vi "test Create Number of Tags.vi"(8 "error in (no error)":errorcluster, 11 "TestCase in":refnum<class "TagTests.lvclass">) -> (0 "error out":errorcluster, 3 "TestCase out":refnum<class "TagTests.lvclass">)   [LabVIEW 2014, in "TagTests.lvclass"]
uses:
  TagTests.lvclass
  <vilib>/addons/_JKI Toolkits/VI Tester/TestCase.llb/TestCase.lvclass
  SPLAT/Tag.lvclass
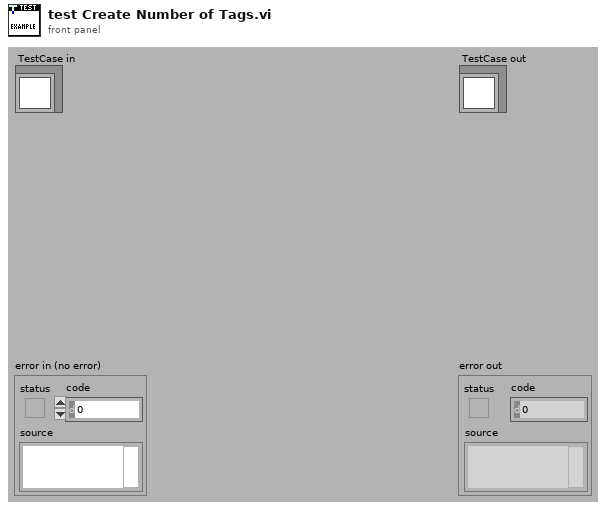
[diagram p1: front panel]
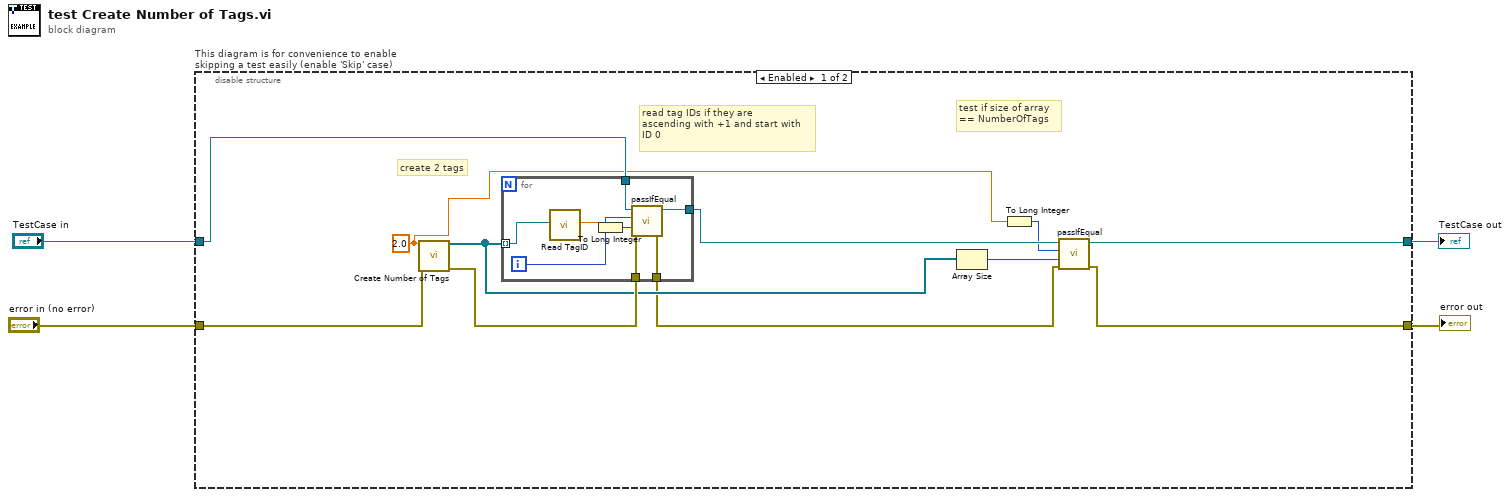
[diagram p0: block diagram]
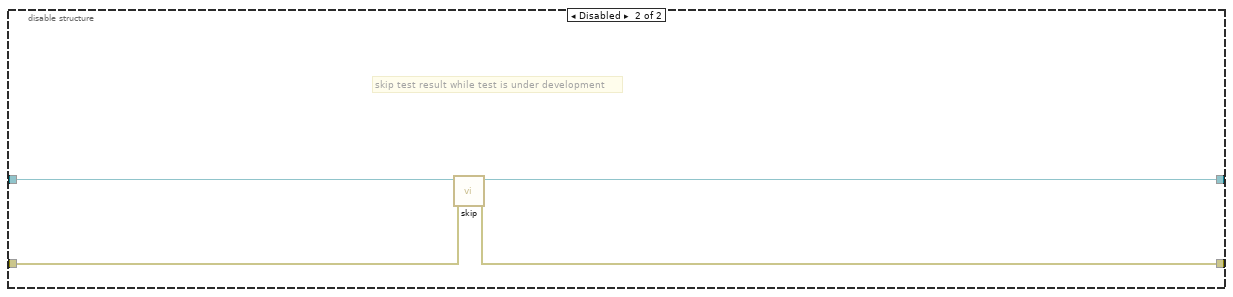
[diagram p2: hidden frame]
diagram:
  n1 = disable-structure "This diagram is for convenience to enable skipping a test easily (enable 'Skip' case)" shown="Enabled" {
    disable-tunnel: "TestCase in" -> [w14 w27]
    disable-tunnel: [w9 w25] -> w1
    disable-tunnel: [w7 w26] -> w3
    disable-tunnel: "error in (no error)" -> [w15 w24]
    frame Enabled {
      w6 = 2.0 ("NumberOfTags")
      # "test if size of array \n== NumberOfTags"
      # "read tag IDs if they are \nascending with +1 and start with\nID 0"
      # "create 2 tags"
      n2 = call "Create Number of Tags.vi"("NumberOfTags"=w6, "error in (no error)"=w15) -> ("TagsArray"=w12:refnum<class "Tag.lvclass">[], "error out"=w13:errorcluster)  [unwired: 12 in]
      n3 = for {
        tunnel: w12 -> [w23] mode=indexing
        tunnel: w14 -> [w21]
        tunnel: [w20] -> w10
        tunnel: w13 -> [w19]
        tunnel: [w18] -> w8
        i -> [w22]
        n4 = call "Read TagID.vi"("Tag in"=w23) -> ("TagID"=w17:dbl)  [unwired: 16 in, 2 out]
        n5 = To Long Integer(number=w17) -> (32bit integer=w16:i32)
        n6 = call-dynamic "passIfEqual.vi"("error in (no error)"=w19, "y"=w16, "x"=w22, "TestCase in"=w21) -> ("error out"=w18:errorcluster, "TestCase out"=w20:refnum<class "TagTests.lvclass">)  [unwired: 6 in]
      }
      n7 = Array Size(array=w12) -> (size(s)=w11:i32)
      n8 = To Long Integer(number=w6) -> (32bit integer=w5:i32)
      n9 = call-dynamic "passIfEqual.vi"("error in (no error)"=w8, "y"=w11, "x"=w5, "TestCase in"=w10) -> ("error out"=w7:errorcluster, "TestCase out"=w9:refnum<class "TagTests.lvclass">)  [unwired: 6 in]
    }
    frame Disabled {
      # "skip test result while test is under development"
      n10 = call <vilib>:"skip.vi"("error in (no error)"=w24, "TestCase in"=w27) -> ("error out"=w26:errorcluster, "TestCase out"=w25:refnum<class "TagTests.lvclass">)  [unwired: 8 in]
    }
  }
  "error out" <- w3
  "TestCase out" <- w1
